vi "Day 18-1.vi"() -> ()   [LabVIEW 2020]
uses:
  SnailNum/SnailNum.lvclass
panel:
  out "Dual Sums":i64[][](array[numeric])
  out "Max Dual Sum":i64
  out "Magnitude":i64
  out "History":string
  out "Final":string
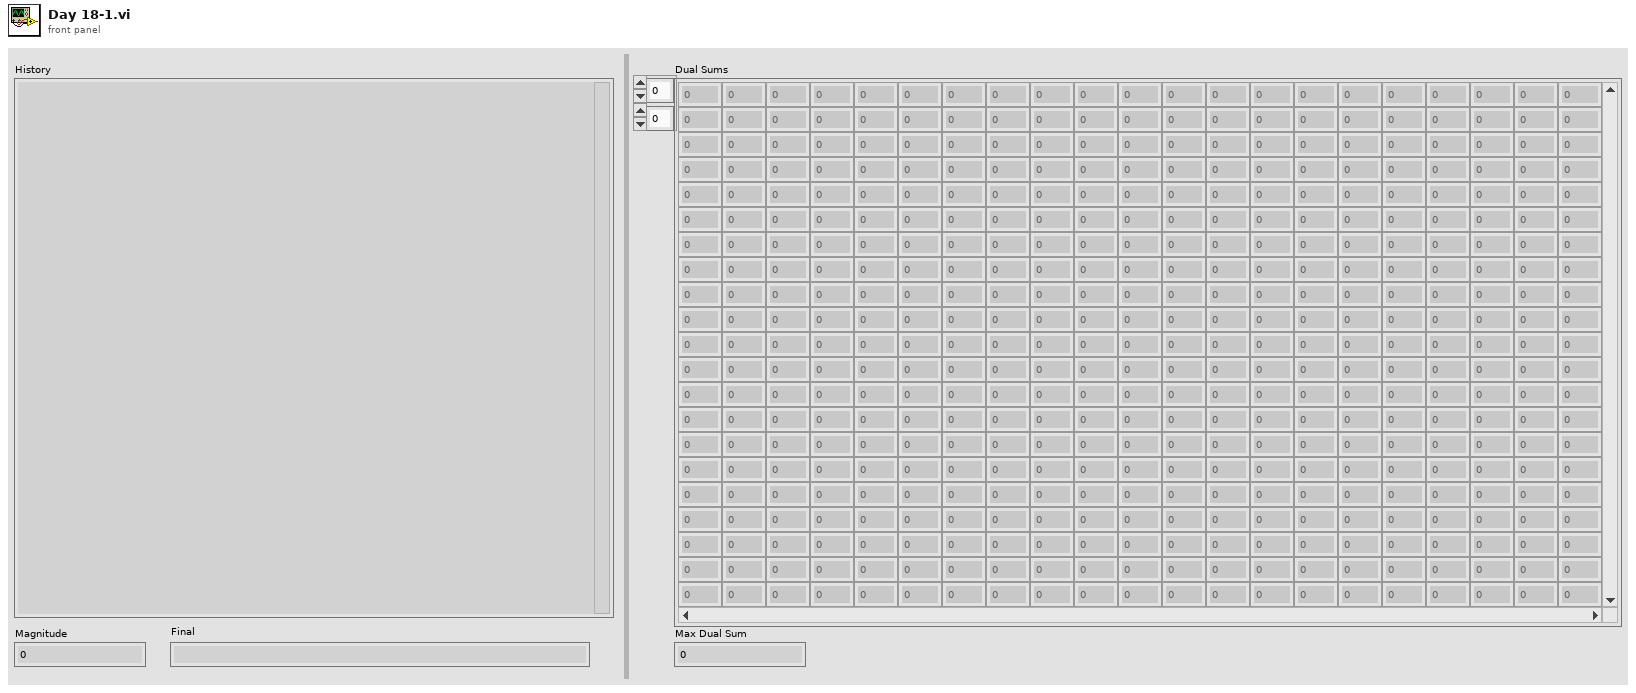
[diagram p1: front panel]
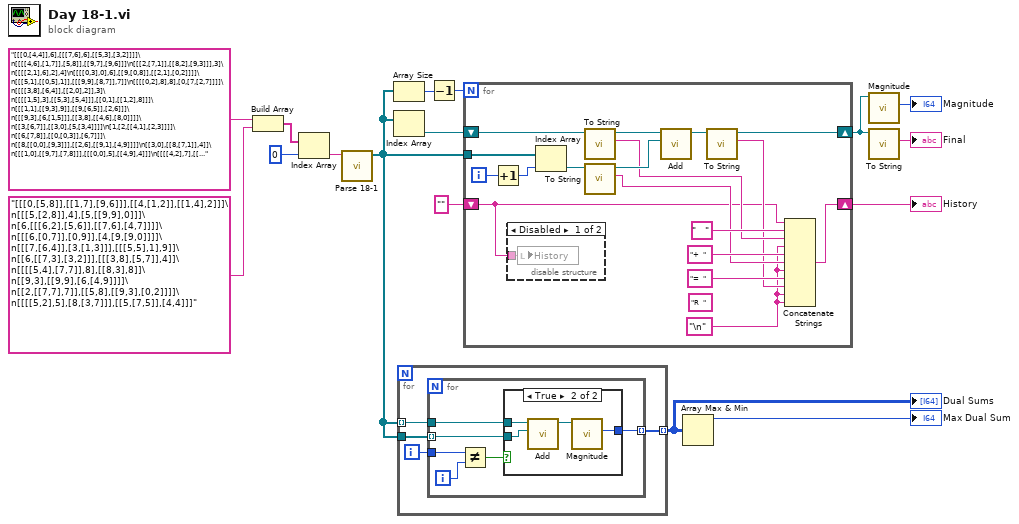
[diagram p0: block diagram]
diagram:
  n1 = Build Array("[[[0,[4,4]],6],[[[7,6],6],[[5,3],[3,2]]]]\n[[[[4,6],[1,7]],[5,8]],[[9,7],[9,6]]]\n[[[2,[7,1]],[[8,2],[9,3]]],3]\n[[[[2,1],6],2],4]\n[[[[0,3],0],6],[[9,[0,8]],[[2,1],[0,2]]]]\n[[[5,1],[[0,5],1]],[[[9,9],[8,7]],7]]\n[[[[0,2],8],8],[0,[7,[2,7]]]]\n[[[[3,8],[6,4]],[[2,0],2]],3]\n[[[[1,5],3],[[5,3],[5,4]]],[[0,1],[[1,2],8]]]\n[[[1,1],[[9,3],9]],[[9,[6,5]],[2,6]]]\n[[[9,3],[6,[1,5]]],[[3,8],[[4,6],[8,0]]]]\n[[3,[6,7]],[[3,0],[5,[3,4]]]]\n[1,[2,[[4,1],[2,3]]]]\n[[6,[7,8]],[[0,[0,3]],[6,7]]]\n[[8,[[0,0],[9,3]]],[[2,6],[[9,1],[4,9]]]]\n[[3,0],[[8,[7,1]],4]]\n[[[1,0],[[9,7],[7,8]]],[[[0,0],5],[[4,9],4]]]\n[[[[4,2],7],[[4,0],0]],[[[5,4],[6,7]],[0,[1,2]]]]\n[[[4,[4,3]],[[1,4],[1,1]]],6]\n[[[0,[5,9]],[[7,4],2]],[[9,1],[4,7]]]\n[[[[5,5],[7,0]],[8,[5,3]]],[[0,[0,2]],[[1,3],[5,8]]]]\n[[9,[[9,9],2]],[[9,6],[[4,7],5]]]\n[[[[8,7],[5,3]],9],[3,[6,9]]]\n[[3,[0,3]],[2,6]]\n[[[2,[7,0]],[6,6]],[[7,0],[[3,8],[8,5]]]]\n[[[2,6],[2,7]],[[3,6],[0,[9,5]]]]\n[[[5,4],1],[5,[[4,9],5]]]\n[[[6,3],6],[[[6,0],0],[[4,0],7]]]\n[[[[4,1],2],[3,[9,0]]],[0,8]]\n[[[2,[3,9]],[[8,3],8]],[[1,[2,2]],[8,[6,4]]]]\n[[[[4,3],[5,2]],0],[9,[5,[7,5]]]]\n[[[3,2],5],[[[6,3],9],[[2,0],[6,7]]]]\n[[[3,9],[[0,6],[0,7]]],[6,[3,2]]]\n[0,0]\n[[[[0,3],9],[8,[3,9]]],[[0,2],[[0,1],[3,7]]]]\n[[0,[4,[3,0]]],[[7,9],[5,[8,7]]]]\n[[2,9],[[0,[2,2]],1]]\n[[[[5,4],[1,7]],6],[2,[[5,3],[7,7]]]]\n[[[[0,4],4],[[6,6],[1,4]]],4]\n[[[[4,8],5],[[6,4],[2,3]]],[9,[[8,6],[4,0]]]]\n[[1,[6,[1,9]]],[3,[[4,2],[1,8]]]]\n[[[[3,7],[5,9]],[[3,8],[3,3]]],[[[7,8],3],[7,3]]]\n[[[[0,4],5],[4,[9,0]]],[3,[[4,1],6]]]\n[[[7,[2,1]],[[1,9],1]],[[[3,4],[8,6]],6]]\n[[[4,1],[5,[8,2]]],[[[1,6],9],[[4,4],2]]]\n[[[7,[6,4]],[[0,1],4]],[[5,2],[[9,5],[9,3]]]]\n[[[4,2],[1,8]],2]\n[[[1,6],5],[8,[2,[2,3]]]]\n[[[[0,2],[5,0]],[7,[0,0]]],[[6,[5,9]],5]]\n[[[7,6],[9,[2,4]]],[[5,[2,6]],2]]\n[[[6,2],4],[[2,9],[[3,0],[4,3]]]]\n[[8,[[6,4],[0,2]]],1]\n[[[4,1],[7,5]],[9,[[2,4],4]]]\n[[[[4,8],[7,5]],[1,[8,5]]],[[3,5],[[9,9],[4,2]]]]\n[[[7,[8,4]],[4,[5,8]]],5]\n[[7,9],[2,[[9,1],[7,1]]]]\n[3,[[[5,8],[4,8]],[5,4]]]\n[[[0,[5,5]],[[5,4],[5,4]]],[[9,6],[[9,4],[6,5]]]]\n[[7,2],[1,[8,[1,7]]]]\n[2,[9,[2,[2,3]]]]\n[[[3,[5,1]],[8,[6,4]]],[[2,8],[[2,2],8]]]\n[[[7,3],[0,4]],[[4,0],[6,[3,4]]]]\n[[4,[2,[2,8]]],[4,[[7,1],9]]]\n[[8,[[6,1],2]],[1,[[1,5],9]]]\n[[0,[2,[9,4]]],[[[7,4],7],8]]\n[[[2,[7,0]],5],[3,[4,4]]]\n[[7,[4,[6,0]]],[[4,7],[[3,7],5]]]\n[[2,[[8,0],[6,1]]],[[6,[6,1]],[3,9]]]\n[[9,0],[[[3,7],0],[[5,8],4]]]\n[6,[[[5,8],8],[3,[4,1]]]]\n[[8,[[9,3],[8,4]]],[4,[8,2]]]\n[[[[8,0],8],[3,7]],[[7,[4,3]],0]]\n[[[7,[2,6]],[8,0]],[4,[[1,3],[4,1]]]]\n[1,[[[4,9],[4,9]],[[7,0],[6,6]]]]\n[9,4]\n[[6,7],4]\n[[2,[5,2]],[[2,4],[[4,6],[5,5]]]]\n[[[5,2],[[5,5],[8,1]]],[[9,[1,6]],3]]\n[[[[4,3],1],[8,9]],6]\n[[[[3,2],[4,5]],4],[[[4,3],[0,0]],[[3,0],1]]]\n[[6,7],[[8,5],[[7,2],4]]]\n[[[[8,1],[5,8]],7],[[[5,2],[4,3]],1]]\n[[2,[[4,9],5]],[1,1]]\n[[9,1],[[[0,8],[1,8]],7]]\n[[9,3],[6,4]]\n[[8,[4,2]],[[7,[7,4]],[[0,9],[6,1]]]]\n[[[[0,5],7],[[7,7],2]],[[2,[5,8]],[9,6]]]\n[[[2,1],[7,[1,3]]],[[2,[7,1]],0]]\n[[[8,[8,4]],[2,[4,3]]],[[2,[5,6]],[[2,0],[7,3]]]]\n[[4,[[4,3],[5,2]]],[1,3]]\n[[5,[5,0]],9]\n[[[2,[7,6]],[1,8]],[[[5,2],2],0]]\n[[2,[2,3]],[[9,8],[[0,1],[3,5]]]]\n[[7,[[3,7],3]],[[[7,6],[4,8]],[[1,7],[8,6]]]]\n[[[0,0],[[6,1],5]],[5,[5,4]]]\n[[2,3],[4,[3,5]]]\n[[8,[7,7]],[8,[4,[8,1]]]]\n[[[[4,0],3],[[0,0],[0,0]]],[[[6,0],4],[[1,7],0]]]\n[[[[6,4],[3,1]],[[2,8],[1,2]]],[4,[[6,5],4]]]\n[[[[5,3],7],[4,[2,6]]],[[6,[4,5]],[1,[9,0]]]]", "[[[0,[5,8]],[[1,7],[9,6]]],[[4,[1,2]],[[1,4],2]]]\n[[[5,[2,8]],4],[5,[[9,9],0]]]\n[6,[[[6,2],[5,6]],[[7,6],[4,7]]]]\n[[[6,[0,7]],[0,9]],[4,[9,[9,0]]]]\n[[[7,[6,4]],[3,[1,3]]],[[[5,5],1],9]]\n[[6,[[7,3],[3,2]]],[[[3,8],[5,7]],4]]\n[[[[5,4],[7,7]],8],[[8,3],8]]\n[[9,3],[[9,9],[6,[4,9]]]]\n[[2,[[7,7],7]],[[5,8],[[9,3],[0,2]]]]\n[[[[5,2],5],[8,[3,7]]],[[5,[7,5]],[4,4]]]") -> (w10:string[])
  n2 = Index Array(array=w10, index=0) -> (element=w9:string)
  n3 = call "Parse 18-1.vi"("Input"=w9) -> ("Numbers"=w4:refnum<class "SnailNum.lvclass">[])  [unwired: 10 in]
  n4 = Array Size(array=w4) -> (size(s)=w16:i32)
  n5 = Index Array(array=w4) -> (element=w15:refnum<class "SnailNum.lvclass">)  [unwired: 1 in]
  n6 = for {
    tunnel: w4 -> [w18] mode=indexing
    tunnel: w4 -> [w19]
    tunnel: [w17] -> w3 mode=indexing
    i -> [w20]
    n7 = for {
      tunnel: w20 -> [w26]
      tunnel: w19 -> [w23] mode=indexing
      tunnel: w18 -> [w22]
      tunnel: [w21] -> w17 mode=indexing
      i -> [w25]
      n8 = Not Equal?(x=w26, y=w25) -> (x != y?=w24:bool)
      n9 = case shown="True" w24 {
        tunnel: w23 -> [_ w29]
        tunnel: w22 -> [_ w30]
        tunnel: [_ w27] -> w21
        frame False {
        }
        frame True {
          n10 = call "Add.vi"("Right"=w29, "Left"=w30) -> ("SnailNum"=w28:refnum<class "SnailNum.lvclass">)  [unwired: 9 in]
          n11 = call "Magnitude.vi"("SnailNum in"=w28) -> ("Magnitude"=w27:i64)  [unwired: 8 in, 2 out]
        }
      }
    }
  }
  "Dual Sums" <- w3
  n12 = Decrement(x=w16) -> (x-1=w14:i32)
  n13 = for {
    N: w14 -> [_]
    tunnel: w4 -> [w48]
    shift-right: [w41] -> w1
    shift-left: w15 -> [w46]
    shift-right: [w35] -> w6
    shift-left: "" -> [w32]
    i -> [w47]
    (unwired) "R  " ("string")
    w33 = "\n"
    n14 = Increment(x=w47) -> (x+1=w44:i32)
    n15 = disable-structure shown="Disabled" {
      disable-tunnel: w32 -> [w49 _]
      frame Disabled {
        n16 = local write "History"(w49) -> ()
      }
      frame Enabled {
      }
    }
    n17 = Index Array(array=w48, index=w44) -> (element=w45:refnum<class "SnailNum.lvclass">)
    n18 = call "To String.vi"("SnailNum in"=w46) -> ("String"=w36:string, "SnailNum out"=w43:refnum<class "SnailNum.lvclass">)  [unwired: 8 in, 1 out]
    n19 = call "To String.vi"("SnailNum in"=w45) -> ("String"=w38:string, "SnailNum out"=w42:refnum<class "SnailNum.lvclass">)  [unwired: 8 in, 1 out]
    n20 = call "Add.vi"("Right"=w42, "Left"=w43) -> ("SnailNum"=w31:refnum<class "SnailNum.lvclass">)  [unwired: 9 in]
    n21 = call "To String.vi"("SnailNum in"=w31) -> ("String"=w34:string, "SnailNum out"=w41:refnum<class "SnailNum.lvclass">)  [unwired: 8 in, 1 out]
    n22 = Concatenate Strings(w32, "   ", w36, w33, "+  " ("string"), w38, w33, "=  " ("string"), w34, w33, w33) -> (w35:string)
  }
  "History" <- w6
  n23 = Array Max & Min(array=w3) -> (max value=→"Max Dual Sum":i64)  [unwired: 3 out]
  n24 = call "Magnitude.vi"("SnailNum in"=w1) -> ("Magnitude"=→"Magnitude":i64)  [unwired: 8 in, 2 out]
  n25 = call "To String.vi"("SnailNum in"=w1) -> ("String"=→"Final":string)  [unwired: 8 in, 2 out]
